vi "CoMP-S TimeStamp Generator.vi"() -> (1 "date/time string":string, 3 "Time hhmmss,units":dbl)   [LabVIEW 2014]
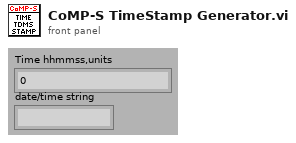
[diagram p1: front panel]
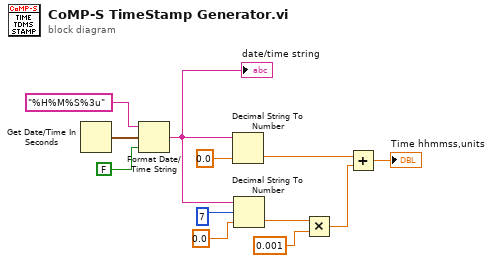
[diagram p0: block diagram]
diagram:
  n1 = Get Date/Time In Seconds() -> (seconds since 1Jan1904=w10:timestamp)
  n2 = Format Date/Time String(time format string (%c)="%H%M%S%3u", seconds (now)=w10, UTC format=FALSE) -> (date/time string=w6:string)
  "date/time string" <- w6
  n3 = Decimal String To Number(string=w6, default (0L)=0.0) -> (number=w2:dbl)  [unwired: 1 in, 1 out]
  n4 = Decimal String To Number(string=w6, offset=7, default (0L)=0.0) -> (number=w5:dbl)  [unwired: 1 out]
  n5 = Multiply(x=w5, y=0.001) -> (x*y=w3:dbl)
  n6 = Add(x=w2, y=w3) -> (x+y=→"Time hhmmss,units":dbl)
